vi "Register Broadcast for Client.vi"(0 "Status":string, 1 "TcpRouter-Client in":refnum<class "TcpRouter-Client.lvclass">, 9 "CSM Name":string="*", 11 "error in (no error)":errorcluster, 12 "Response Timeout(5000ms)":i32=5000, 13 "Priority (No Change)":T1) -> (4 "CSM Name(dup)":string, 15 "error out":errorcluster)   [LabVIEW 2020, in "CSM-TCP-Router.lvlib" / "TcpRouter-Client.lvclass"]
uses:
  TcpRouter-Client.lvclass
  <userlib>/_NEVSTOP/Communicable State Machine(CSM)/AdvanceAPI/CSM - Broadcast Message Type.ctl
  TcpRouter-Client.lvclass/TcpRouter-Client.ctl
  _support/tcp-msg type.ctl
  5c4b9d63-4fec-4512-8845-8d145ac2895f.vi
  <userlib>/_NEVSTOP/Communicable State Machine(CSM)/AdvanceAPI/CSM - Revert Arguments-Safe String.vi
  <userlib>/_NEVSTOP/Communicable State Machine(CSM)/AdvanceAPI/CSM - Keywords.vi
  <userlib>/_NEVSTOP/Communicable State Machine(CSM)/_Polymophic/Build Register Message.vi
  <userlib>/_NEVSTOP/Communicable State Machine(CSM)/_Shared/Trim Single-line Text.vi
  <userlib>/_NEVSTOP/Communicable State Machine(CSM)/Communicable State Machine.lvlib
  CSM-TCP-Router.lvlib
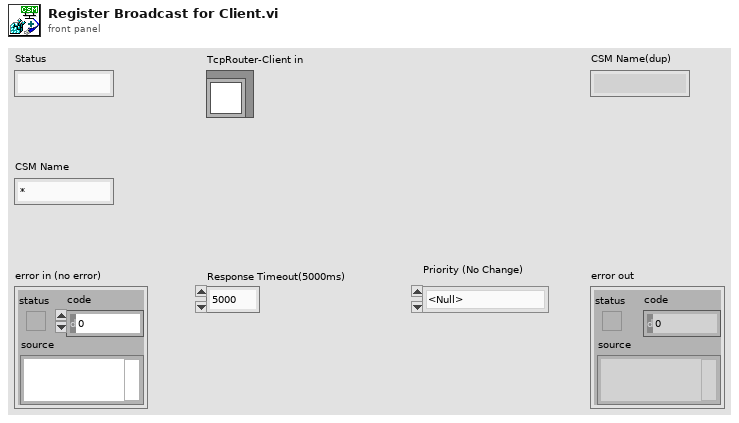
[diagram p1: front panel]
types:
  T1 = typedef "Communicable State Machine.lvlib/CSM - Broadcast Message Type.ctl" = enum16{"<Null>", "Status", "Interrupt"}
  T2 = typedef "CSM-TCP-Router.lvlib/tcp-msg type.ctl" = enum8{"info", "error", "cmd", "cmd-resp", "resp", "async-resp", "status", "interrupt"}
  T3 = typedef "CSM-TCP-Router.lvlib/TcpRouter-Client.lvclass/Def-TCP-Router PUB-SUB.ctl" = cluster{"STATUS":refnum<k5>, "StatusQueue":refnum<queue>}
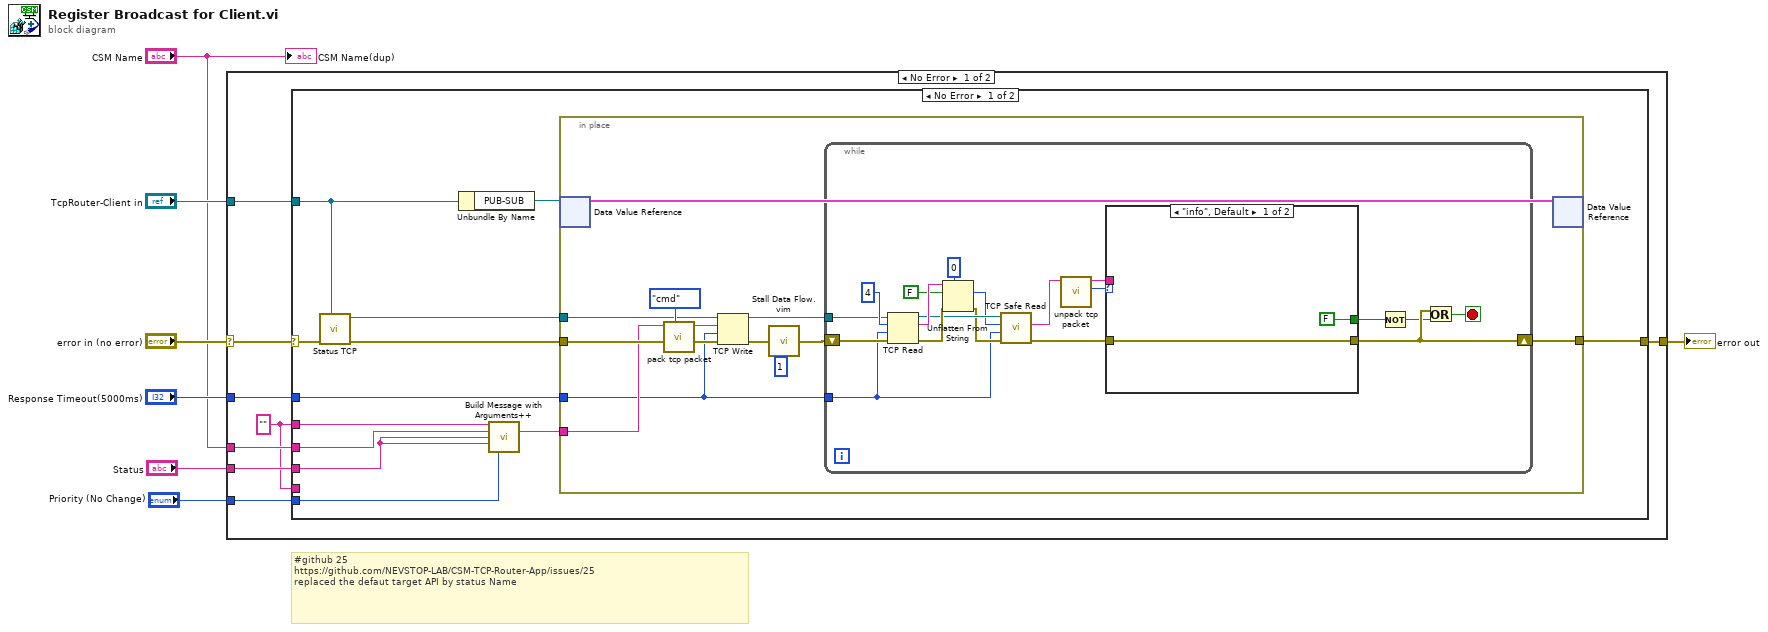
[diagram p0: block diagram]
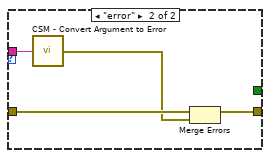
[diagram p2: hidden frame]
diagram:
  # "#github 25\nhttps://github.com/NEVSTOP-LAB/CSM-TCP-Router-App/issues/25\nreplaced the defaut target API by status Name"
  n1 = case shown="No Error" "error in (no error)" {
    selector: "error in (no error)" -> [w15 w66]
    tunnel: [w14 w66] -> w6
    tunnel: "TcpRouter-Client in" -> [w13 _]
    tunnel: "Response Timeout(5000ms)" -> [w12 _]
    tunnel: "CSM Name" -> [w11 _]
    tunnel: "Status" -> [w10 _]
    tunnel: "Priority (No Change)" -> [w8 _]
    frame No Error {
      w9 = "" ("Source CSM Name (* as Default)")
      n2 = case shown="No Error" w15 {
        selector: w15 -> [w27 w65]
        tunnel: [w25 w65] -> w14
        tunnel: w13 -> [w24 _]
        tunnel: w12 -> [w17 _]
        tunnel: w9 -> [w21 _]
        tunnel: w11 -> [w22 _]
        tunnel: w10 -> [w16 _]
        tunnel: w9 -> [_ _]
        tunnel: w8 -> [w20 _]
        frame No Error {
          n3 = call "Status TCP.vi"("TcpRouter-Client in"=w24, "error in (no error)"=w27) -> ("error out"=w19:errorcluster, "connection ID"=w18:refnum<k5>)  [unwired: 8 in]
          n4 = Unbundle By Name(w24) -> ("PUB-SUB"=w23:refnum<data-value>)
          n5 = call-poly <userlib>:"Build Message with Arguments++.vi"("Target CSM"=w21, "Source CSM (* as Default)"=w22, "Status"=w16, "API (If \"\", Same As \"Status\")"=w16, "Priority (No Change)"=w20) -> ("CSM Message String"=w26:string)  [unwired: 10 in]
          n6 = in-place {
            in-place-border: w19 -> [w37]
            in-place-border: w18 -> [w36]
            in-place-border: w26 -> [w35]
            in-place-border: [w30] -> w25
            in-place-border: w17 -> [w29]
            n7 = in-place-dvr #1(w23) -> (w28:T3)  [unwired: 1 out]
            n8 = call "pack tcp packet.vi"("tcp-message-type"=tcp-msg_type."cmd", "String"=w35) -> ("TCP Pack"=w39:string)  [unwired: 9 in]
            n9 = TCP Write(connection ID=w36, data in=w39, error in (no error)=w37, 9:w29) -> (connection ID out=w32:refnum<k5>, error out=w34:errorcluster)  [unwired: 1 out]
            n10 = call "Stall Data Flow.vim"("value in"=w34, "milliseconds to wait"=u32 1) -> ("value out"=w31:errorcluster)  [unwired: 1 out]
            n11 = while {
              tunnel: w32 -> [w49]
              shift-right: [w44] -> w30
              shift-left: w31 -> [w48]
              tunnel: w29 -> [w43]
              stop <- w42 stop-if-true
              n12 = TCP Read(connection ID=w49, bytes to read=4, error in (no error)=w48, 9:w43) -> (connection ID out=w56:refnum<k5>, data out=w57:string, error out=w58:errorcluster)  [unwired: 1 in]
              n13 = Unflatten From String(type=0, binary string=w57, data includes array or string size? (T)=FALSE, error in (no error)=w58) -> (value=w54:i32, error out=w53:errorcluster)  [unwired: 2 out]
              n14 = call "TCP Safe Read.vi"("error in (no error)"=w53, "timeout ms (25000)"=w43, "bytes to read"=w54, "TCP Network Connection in"=w56) -> ("error out"=w46:errorcluster, "String"=w55:string)  [unwired: 5 in, 1 out]
              n15 = call "unpack tcp packet.vi"("TCP Pack"=w55) -> ("tcp-message-type"=w47:T2, "String"=w45:string)  [unwired: 9 in]
              n16 = case shown="\"info\", Default" w47 {
                tunnel: w46 -> [w60 w64]
                tunnel: [w60 w62] -> w44
                tunnel: w45 -> [_ w63]
                tunnel: [FALSE _] -> w41
                frame "info", Default {
                }
                frame "error" {
                  n17 = call <userlib>:"CSM - Convert Argument to Error.vi"("Argument"=w63) -> ("Error"=w61:errorcluster)  [unwired: 4 in]
                  n18 = Merge Errors(w64, w61) -> (w62:errorcluster)
                }
              }
              n19 = Not(x=w41) -> (.not. x?=w40:bool)
              n20 = Or(x=w44, y=w40) -> (x .or. y?=w42:bool)
            }
            n21 = in-place-dvr #1(w28) -> ()  [unwired: 2 out]
          }
        }
        frame Error {
        }
      }
    }
    frame Error {
    }
  }
  "error out" <- w6
  "CSM Name(dup)" <- "CSM Name"
